vi "Write Tag Data.vi"(8 "error in (no error)":errorcluster, 11 "data":waveform(dbl)[](array[waveform])) -> (0 "error out":errorcluster)   [LabVIEW 2018, in "DAQ.lvlib" / "DAQ Write.lvlib"]
uses:
  DAQ/DAQ Write.lvlib
  Tag VIs/Tag FGV Operation Enum.ctl
  <vilib>/Analysis/baseanly.llb/Mean (DBL).vi
  Shared Variables/Dynamic Shared Variables.lvlib
  <vilib>/Analysis/NI_AALBase.lvlib
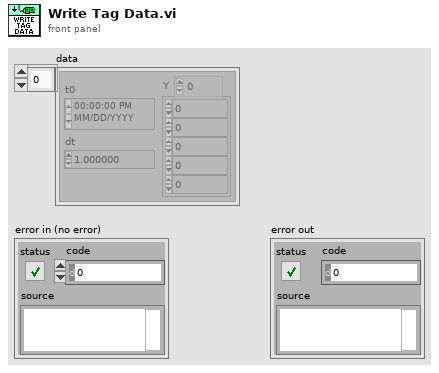
[diagram p1: front panel]
types:
  T1 = typedef "Tag FGV Operation Enum.ctl" = enum16{"Init", "Set Notification Queue", "Create Tag", "Commit", "Write Tag (Numeric)", "Write Tag (Boolean)", "Read All Tags", "Read One Tag", "Delete Tag Category", "Set Alarm Parameters (Numeric)", "Set Alarm Parameters (Boolean)", "Enable All Alarms", "Disable All Alarms", "Delete All Tags", "Read Alarms", "Ack Alarm", "Read Alarm Parameters (Numeric)", "Read Alarm Parameters (Boolean)"}
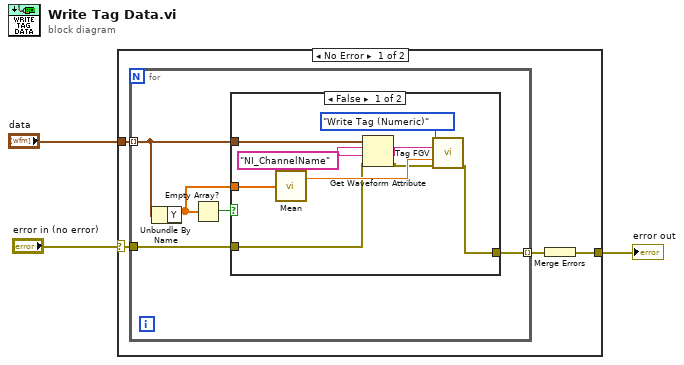
[diagram p0: block diagram]
diagram:
  n1 = case shown="No Error" "error in (no error)" {
    selector: "error in (no error)" -> [w6 w23]
    tunnel: [w4 w23] -> w2
    tunnel: "data" -> [w7 _]
    frame No Error {
      n2 = for {
        tunnel: w7 -> [w12] mode=indexing
        tunnel: w6 -> [w9]
        tunnel: [w8] -> w5 mode=indexing
        n3 = Unbundle By Name(w12) -> ("Y"=w10:dbl[])
        n4 = Empty Array?(array=w10) -> (empty?=w11:bool)
        n5 = case shown="False" w11 {
          tunnel: w12 -> [w18 _]
          tunnel: w10 -> [w17 _]
          tunnel: w9 -> [w14 w22]
          tunnel: [w13 w22] -> w8
          frame False {
            w20 = "NI_ChannelName" ("name")
            n6 = call-poly <vilib>:"Mean.vi"("X"=w17) -> ("mean"=w16:dbl)  [unwired: 1 out]
            n7 = Get Waveform Attribute(4:w14, 5:w20, 6:w20, 7:w18) -> (0:w15:errorcluster, 1:w19:string)  [unwired: 2 out]
            n8 = call "Tag FGV.vi"("Operation"=Tag_FGV_Operation_Enum."Write Tag (Numeric)", "Tag Name"=w19, "Data"=w16, "error in (no error)"=w15) -> ("error out"=w13:errorcluster)  [unwired: 4 in, 7 out]
          }
          frame True {
          }
        }
      }
      n9 = Merge Errors(w5) -> (w4:errorcluster)
    }
    frame Error {
    }
  }
  "error out" <- w2
